vi "判断时间正常.vi"(8 "error in (no error)":errorcluster caption="错误输入（无错误）") -> (0 "error out":errorcluster caption="错误输出", 3 "时间正常":bool)   [LabVIEW 2014]
panel:
  out "t1":dbl format="%#.6f"
  out "t2":dbl format="%#.6f"
  out "双精度浮点数":dbl
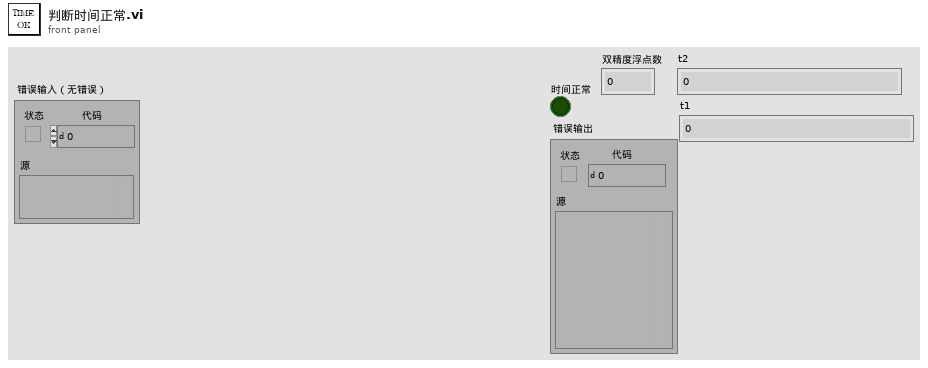
[diagram p1: front panel]
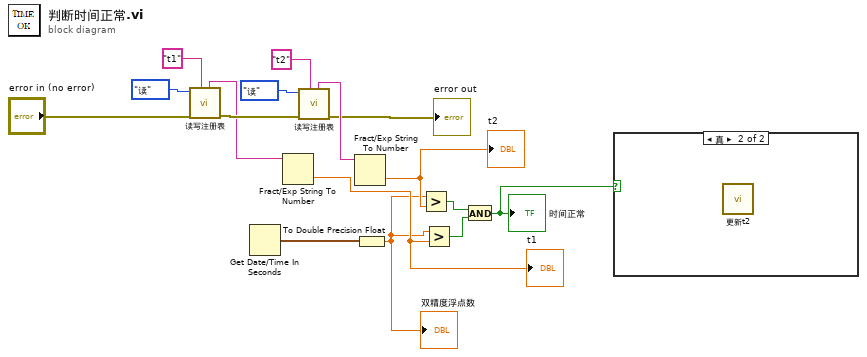
[diagram p0: block diagram]
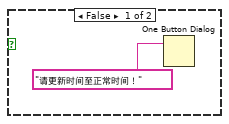
[diagram p2: hidden frame]
diagram:
  n1 = call "读写注册表.vi"("键名称"="t1", "error in (no error)"="error in (no error)", "读/写"=enum16{"读", "写"}."读") -> ("error out"=w12:errorcluster, "键内容"=w11:string)  [unwired: 7 in]
  n2 = Get Date/Time In Seconds() -> (seconds since 1Jan1904=w9:timestamp)
  n3 = Fract/Exp String To Number(string=w11) -> (number=w7:dbl)  [unwired: 3 in, 1 out]
  "t1" <- w7
  n4 = call "读写注册表.vi"("键名称"="t2", "error in (no error)"=w12, "读/写"=enum16{"读", "写"}."读") -> ("error out"=→"error out":errorcluster, "键内容"=w10:string)  [unwired: 7 in]
  n5 = Fract/Exp String To Number(string=w10) -> (number=w8:dbl)  [unwired: 3 in, 1 out]
  "t2" <- w8
  n6 = To Double Precision Float(number=w9) -> (double precision float=w6:dbl)
  "双精度浮点数" <- w6
  n7 = Greater?(x=w6, y=w8) -> (0:w5:bool)
  n8 = Greater?(x=w6, y=w7) -> (0:w4:bool)
  n9 = And(x=w5, y=w4) -> (x .and. y?=w1:bool)
  "时间正常" <- w1
  n10 = case shown="真" w1 {
    frame False {
      n11 = One Button Dialog(message="请更新时间至正常时间！" ("消息")) -> ()  [unwired: 1 in, 1 out]
    }
    frame True {
      n12 = call "更新t2.vi"() -> ()  [unwired: 11 in, 1 out]
    }
  }
